vi "SaveDataLog.vi"(7 "Data Log Path":path, 8 "error in (no error)":errorcluster, 11 "Offset":cluster{"Angle":sgl, "AngEle":sgl, "RCS":sgl}[](array[cluster])) -> (0 "error out":errorcluster)   [LabVIEW 2024]
uses:
  <vilib>/Utility/file.llb/Write Delimited Spreadsheet (string).vi
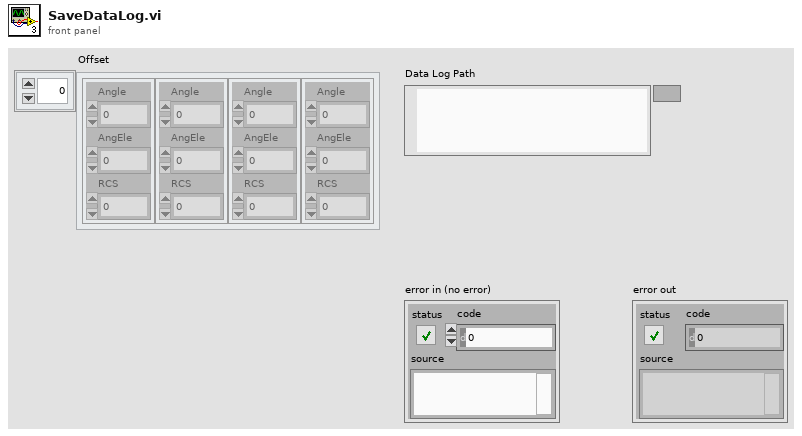
[diagram p1: front panel]
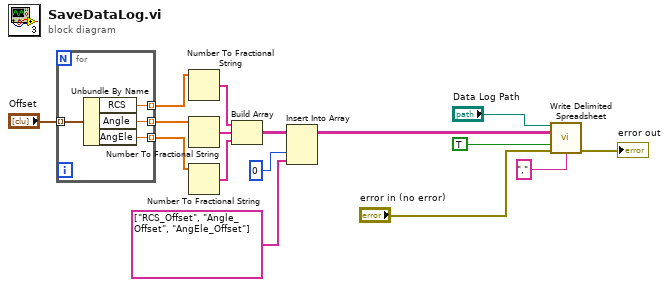
[diagram p0: block diagram]
diagram:
  n1 = for {
    tunnel: "Offset" -> [w20] mode=indexing
    tunnel: [w19] -> w12 mode=indexing
    tunnel: [w18] -> w11 mode=indexing
    tunnel: [w17] -> w10 mode=indexing
    n2 = Unbundle By Name(w20) -> ("RCS"=w19:sgl, "Angle"=w18:sgl, "AngEle"=w17:sgl)
  }
  n3 = Number To Fractional String(number=w12) -> (F-format string=w9:string[])  [unwired: 3 in]
  n4 = Number To Fractional String(number=w11) -> (F-format string=w8:string[])  [unwired: 3 in]
  n5 = Number To Fractional String(number=w10) -> (F-format string=w7:string[])  [unwired: 3 in]
  n6 = Build Array(w9, w8, w7) -> (w6:string[][])
  n7 = Insert Into Array(array=w6, index (col)=0 ("disabled index (col)"), new element=string[] ["RCS_Offset", "Angle_Offset", "AngEle_Offset"]) -> (w3:string[][])  [unwired: 1 in]
  n8 = call-poly <vilib>:"Write Delimited Spreadsheet.vi"("file path (dialog if empty)"="Data Log Path", "2D data"=w3, "append to file? (new file:F)"=TRUE, "error in (no error)"="error in (no error)", "delimiter (\\t)"="," ("delimiter (\\t)")) -> ("error out"=→"error out":errorcluster)  [unwired: 9 in, 1 out]
